vi "ConfigFileReader.vi"() -> ()   [LabVIEW 2011]
uses:
  <vilib>/Utility/config.llb/NI_LVConfig.lvlib
  <vilib>/Utility/config.llb/Read Key (Double).vi
panel:
  out "appended array":refnum<vi>[](array[refnum])
  out "Label.Text":string
  out "Guidage":T1
  out "Camera":T2={"Naxis1"=142, "Naxis2"=99, "PixScale1"=0.323, "PixScale2"=0.323, "ROIHeight"=0, "ROIWidth"=0, "ROIHeight 2"=0, "ROIWidth 2"=0, "Binning"=0} {"Binning" items=["1 x 1"=1, "2 x 2"=2, "4 x 4"=4, "5 x 5"=5]; "PixScale2" format="%.4f"; "PixScale1" format="%.4f"}
  out "Variables":T3={"a3_focus"=3.3333e-05, "a1_focus"=345622.0, "a2_focus"=3.3333e-05, "k0_focus"=3.3333e-05, "k1_focus"=3.3333e-05, "dflt-EQX"=2008.731741} {"dflt-EQX" format="%.6f"; "k1_focus" format="%.4e"; "k0_focus" format="%.4e"; "a2_focus" format="%.4e"; "a1_focus" min=0.0 max=500000.0 step=10000.0; "a3_focus" format="%.4e"}
  out "properties.ini":path=path "C:/BonOMM/BonOMM 7.1/BonOMM 7.1.vi" caption="Fichier de Configuration Système"
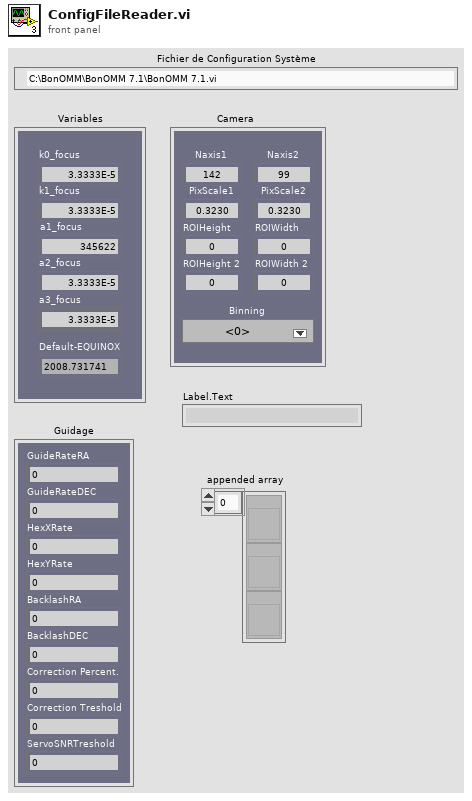
[diagram p1: front panel]
types:
  T1 = cluster{"BacklashRA":dbl, "RateRA":dbl, "HexXRate":dbl, "HexYRate":dbl, "BacklashDEC":dbl, "RateDEC":dbl, "CorrTreshold":dbl, "Corr%":dbl, "SNRtreshold":dbl}
  T2 = cluster{"Naxis1":u16, "Naxis2":u16, "PixScale1":dbl, "PixScale2":dbl, "ROIHeight":u16, "ROIWidth":u16, "ROIHeight 2":u16, "ROIWidth 2":u16, "Binning":u16}
  T3 = cluster{"a3_focus":dbl, "a1_focus":dbl, "a2_focus":dbl, "k0_focus":dbl, "k1_focus":dbl, "dflt-EQX":dbl}
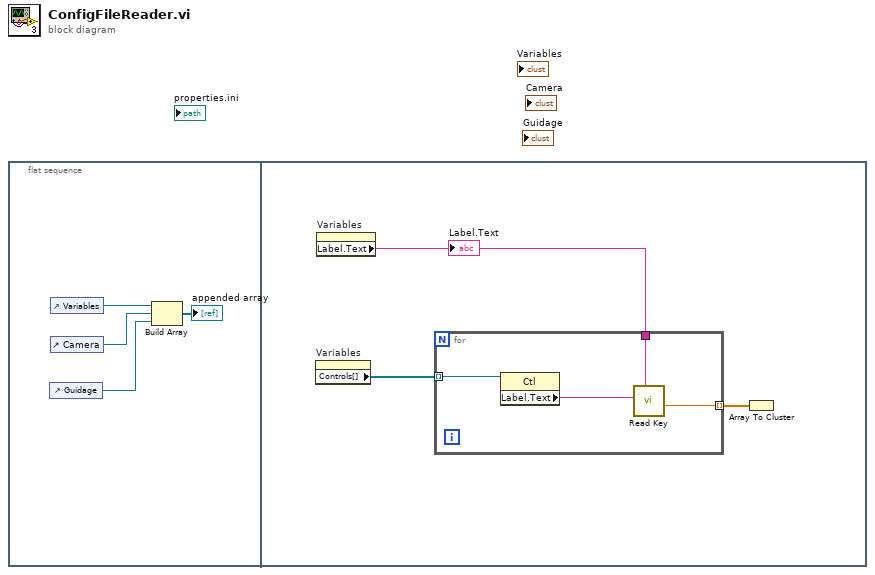
[diagram p0: block diagram]
diagram:
  n1 = flat-sequence {
    frame #0 {
      n2 = control-ref of="Guidage"() -> (w2:refnum<vi>)
      n3 = control-ref of="Variables"() -> (w3:refnum<vi>)
      n4 = control-ref of="Camera"() -> (w4:refnum<vi>)
      n5 = Build Array(w3, w4, w2) -> (→"appended array":refnum<vi>[])
    }
    frame #1 {
      n6 = property on="Variables" class="Clust (strict)"() -> ("Controls[]"=w7:refnum<vi>[])  [unwired: 2 in, 2 out]
      n7 = property on="Variables" class="Clust (strict)"() -> ("Label.Text"=w6:string)  [unwired: 2 in, 2 out]
      "Label.Text" <- w6
      n8 = for {
        tunnel: w7 -> [w11] mode=indexing
        tunnel: w6 -> [w9]
        tunnel: [w8] -> w5 mode=indexing
        n9 = property class="Ctl"(reference=w11) -> ("Label.Text"=w10:string)  [unwired: 1 in, 2 out]
        n10 = call-poly <vilib>:"Read Key.vi"("section"=w9, "key"=w10) -> ("value"=w8:dbl)  [unwired: 6 in, 3 out]
      }
      n11 = Array To Cluster(array=w5) -> ()  [unwired: 1 out]
    }
  }
